vi "AssetMgrCreateOrUpdateCamerasRequest_Parse.vi"(8 "error in (no error)":errorcluster, 11 "Message":T8) -> (0 "error out":errorcluster, 1 "Body":T1, 2 "Header":T7, 3 "AssetMgrCreateOrUpdateCamerasRequest":T6)   [LabVIEW 2017]
uses:
  <vilib>/addons/InsightCM/MessageBus/Base/controls/Message.ctl
  <vilib>/addons/InsightCM/MessageBus/Base/controls/MessageHeader.ctl
  <vilib>/addons/InsightCM/MessageBus/Base/controls/KeyValuePair.ctl
  <vilib>/addons/InsightCM/MessageBus/MessageLibrary/AssetManager/controls/AssetMgrCreateOrUpdateCamerasRequest.ctl
  <vilib>/addons/InsightCM/MessageBus/MessageLibrary/AssetManager/controls/AssetMgrCreateOrUpdateCamerasRequestBody.ctl
  <vilib>/addons/InsightCM/MessageBus/Base/controls/Camera.ctl
  <vilib>/addons/InsightCM/MessageBus/Base/controls/Trigger.ctl
  <vilib>/addons/InsightCM/MessageBus/Base/controls/Condition.ctl
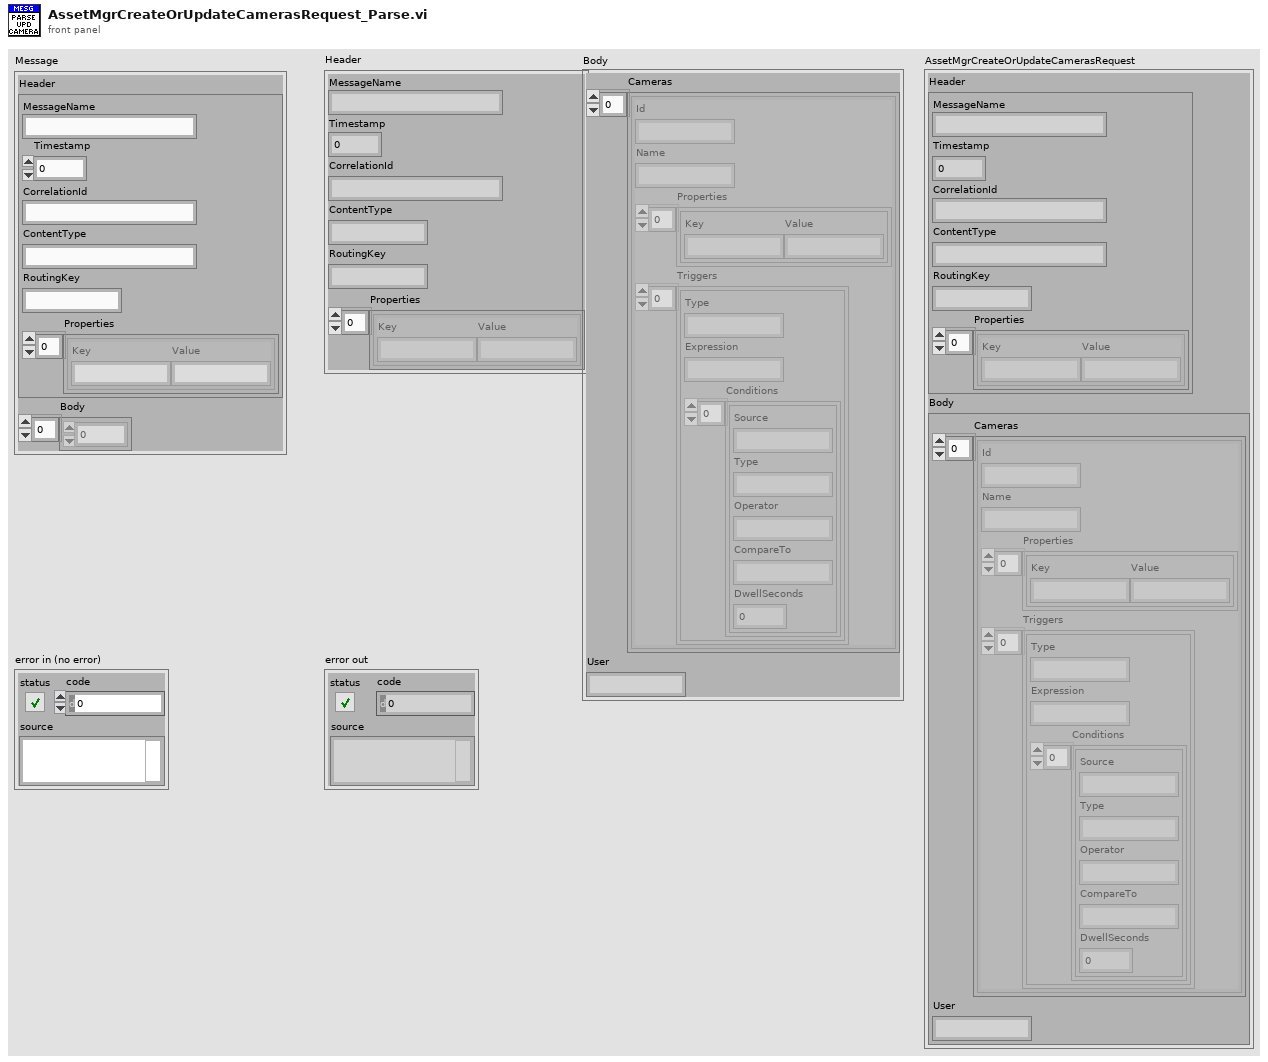
[diagram p1: front panel]
types:
  T1 = typedef "AssetMgrCreateOrUpdateCamerasRequestBody.ctl" = cluster{"Cameras":T2[], "User":string}
  T2 = typedef "Camera.ctl" = cluster{"Id":string, "Name":string, "Properties":T3[], "Triggers":T4[]}
  T3 = typedef "KeyValuePair.ctl" = cluster{"Key":string, "Value":string}
  T4 = typedef "Trigger.ctl" = cluster{"Type":string, "Expression":string, "Conditions":T5[]}
  T5 = typedef "Condition.ctl" = cluster{"Source":string, "Type":string, "Operator":string, "CompareTo":string, "DwellSeconds":dbl}
  T6 = typedef "AssetMgrCreateOrUpdateCamerasRequest.ctl" = cluster{"Header":T7, "Body":T1}
  T7 = typedef "MessageHeader.ctl" = cluster{"MessageName":string, "Timestamp":i64, "CorrelationId":string, "ContentType":string, "RoutingKey":string, "Properties":T3[]}
  T8 = typedef "Message.ctl" = cluster{"Header":T7, "Body":u8[]}
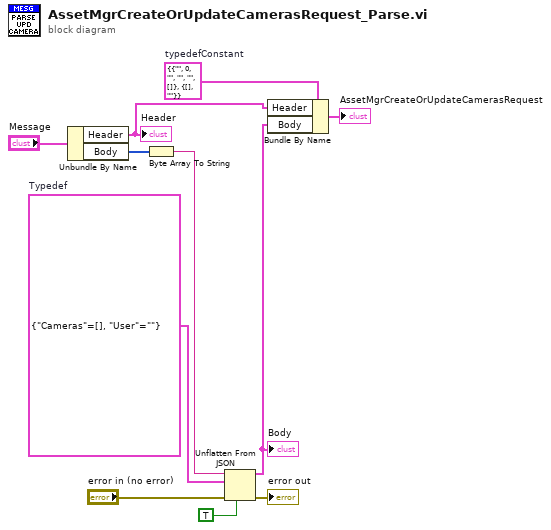
[diagram p0: block diagram]
diagram:
  w3 = T6 {"Header"={"MessageName"="", "Timestamp"=0, "CorrelationId"="", "ContentType"="", "RoutingKey"="", "Properties"=[]}, "Body"={"Cameras"=[], "User"=""}}  # typedefConstant
  w7 = T1 {"Cameras"=[], "User"=""}  # Typedef
  n1 = Unbundle By Name("Message") -> ("Header"=w9:T7, "Body"=w1:u8[])
  "Header" <- w9
  n2 = Byte Array To String(unsigned byte array=w1) -> (string=w6:string)
  n3 = Unflatten From JSON(JSON string=w6, type and defaults=w7, default null elements? (F)=TRUE, error in (no error)="error in (no error)") -> (value=w5:T1, error out=→"error out":errorcluster)  [unwired: 3 in]
  "Body" <- w5
  n4 = Bundle By Name(cluster=w3, "Header"=w9, "Body"=w5) -> (→"AssetMgrCreateOrUpdateCamerasRequest":T6)
